vi "Example Modbus Slave.vi"() -> ()   [LabVIEW 2010]
uses:
  C:/tf/play/labview/Tinkerforge.dll
  Tinkerforge.dll
panel:
  out "registerValue":i32
  out "registerAddress":i64
  out "message":string
  out "requestID":u8
  in  "stop":bool
  in  "uid":string="amb"
  in  "port":i32=4223
  in  "host":string="localhost"
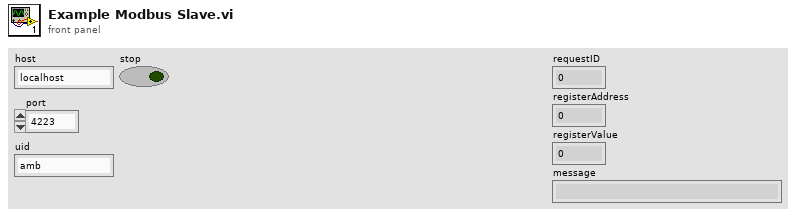
[diagram p1: front panel]
types:
  T1 = cluster{"requestID":u8, "registerAddress":i64, "registerValue":i32}
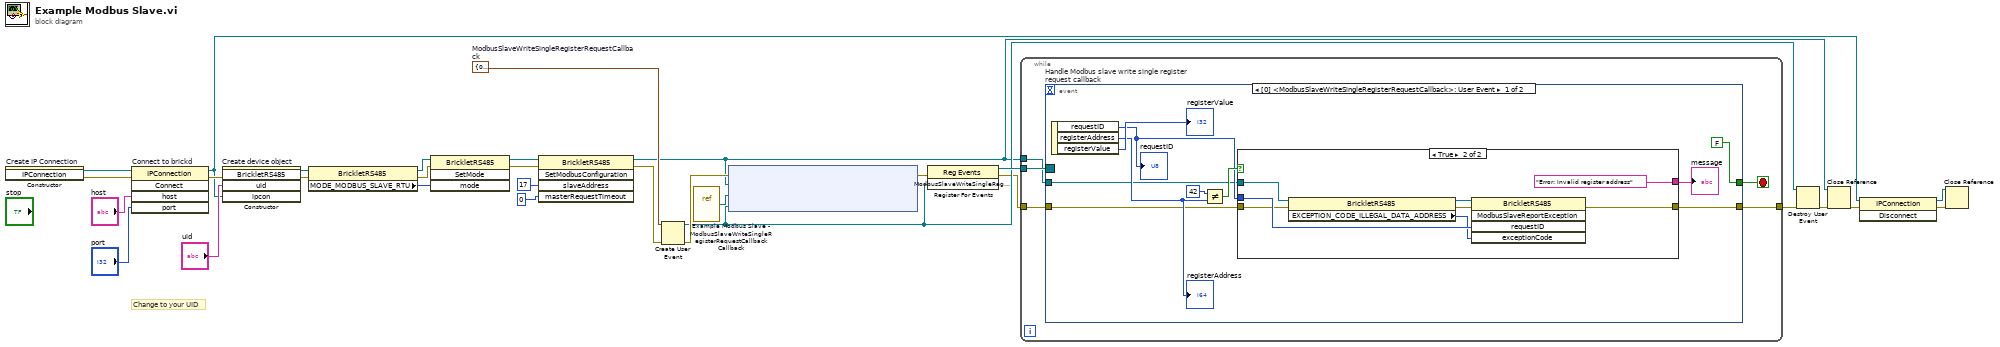
[diagram p0: block diagram]
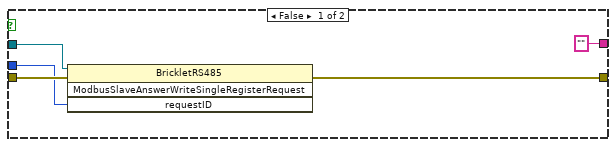
[diagram p2: hidden frame]
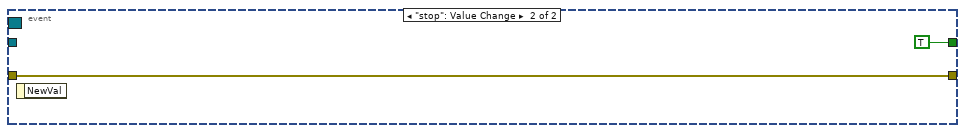
[diagram p3: hidden frame]
diagram:
  w14 = T1 {"requestID"=0, "registerAddress"=0, "registerValue"=0}  # ModbusSlaveWriteSingleRegisterRequestCallback
  # "Change to your UID"
  n1 = constructor on="Create IP Connection" class="IPConnection"() -> (reference out=w30:refnum<k24>, error out=w15:errorcluster)  [unwired: 3 in, 1 out]
  n2 = invoke on="Connect to brickd" class="IPConnection" method="Connect"(reference=w30, error in=w15, "host"="host", "port"="port") -> (reference out=w23:refnum<k24>, error out=w26:errorcluster)  [unwired: 1 in, 3 out]
  n3 = constructor on="Create device object" class="BrickletRS485"(error in=w26, "uid"="uid", "ipcon"=w23) -> (reference out=w13:refnum<k24>, error out=w12:errorcluster)  [unwired: 2 in, 3 out]
  n4 = property class="BrickletRS485"(reference=w13, error in=w12) -> (reference out=w10:refnum<k24>, error out=w11:errorcluster, "MODE_MODBUS_SLAVE_RTU"=w9:u8)
  n5 = invoke class="BrickletRS485" method="SetMode"(reference=w10, error in=w11, "mode"=w9) -> (reference out=w8:refnum<k24>, error out=w6:errorcluster)  [unwired: 1 in, 2 out]
  n6 = invoke class="BrickletRS485" method="SetModbusConfiguration"(reference=w8, error in=w6, "slaveAddress"=u8 17, "masterRequestTimeout"=i64 0) -> (reference out=w1:refnum<k24>, error out=w7:errorcluster)  [unwired: 1 in, 3 out]
  n7 = Create User Event(user event datatype=w14, error in=w7) -> (user event=w17:refnum<user-event>, error out=w21:errorcluster)
  n8 = vi-ref "Example Modbus Slave - ModbusSlaveWriteSingleRegisterRequestCallback Callback.vi"() -> ("vi reference"=w2:refnum<vi>)
  n9 = node ("Register Event Callback")(w21, w1, w2, w17) -> (w20:errorcluster)  [unwired: 1 in, 1 out]
  n10 = register-events(error in=w20, w17) -> (reference out=w19:refnum<event-registration>, error out=w3:errorcluster)  [unwired: 1 in]
  n11 = while {
    tunnel: w19 -> [w32]
    tunnel: [w35] -> w18
    tunnel: w3 -> [w34]
    tunnel: w1 -> [w31]
    stop <- w33 stop-if-true
    n12 = event "Handle Modbus slave write single register request callback" shown="[0] <ModbusSlaveWriteSingleRegisterRequestCallback>: User Event" {
      selector: w32 -> [_ _]
      dyn-events: _ -> [_ _]
      timeout: _ -> [_ _]
      tunnel: [w38 w59] -> w35
      tunnel: w34 -> [w39 w59]
      tunnel: [FALSE TRUE] -> w33
      tunnel: w31 -> [w36 _]
      event User Event {
        n13 = event-data() -> ("requestID"=w37:u8, "registerAddress"=w43:i64, "registerValue"=→"registerValue":i32)  [unwired: 1 in]
        "requestID" <- w37
        "registerAddress" <- w43
        n14 = Not Equal?(x=i64 42, y=w43) -> (x != y?=w41:bool)
        n15 = case shown="True" w41 {
          tunnel: ["" ("f") "Error: Invalid register address"] -> w40
          tunnel: w39 -> [w48 w54]
          tunnel: [w46 w57] -> w38
          tunnel: w37 -> [w47 w56]
          tunnel: w36 -> [w49 w55]
          frame False {
            n16 = invoke class="BrickletRS485" method="ModbusSlaveAnswerWriteSingleRegisterRequest"(reference=w49, error in=w48, "requestID"=w47) -> (error out=w46:errorcluster)  [unwired: 1 in, 3 out]
          }
          frame True {
            n17 = property class="BrickletRS485"(reference=w55, error in=w54) -> (reference out=w52:refnum<k24>, error out=w53:errorcluster, "EXCEPTION_CODE_ILLEGAL_DATA_ADDRESS"=w51:i16)
            n18 = invoke class="BrickletRS485" method="ModbusSlaveReportException"(reference=w52, error in=w53, "requestID"=w56, "exceptionCode"=w51) -> (error out=w57:errorcluster)  [unwired: 1 in, 4 out]
          }
        }
        "message" <- w40
      }
      event "stop": Value Change {
        n19 = event-data() -> ()  [unwired: 1 in, 1 out]
      }
    }
  }
  n20 = Destroy User Event(user event=w17, error in=w18) -> (error out=w16:errorcluster)
  n21 = Close Reference(reference=w1, error in (no error)=w16) -> (error out=w25:errorcluster)
  n22 = invoke class="IPConnection" method="Disconnect"(reference=w23, error in=w25) -> (reference out=w22:refnum<k24>, error out=w24:errorcluster)  [unwired: 1 in, 1 out]
  n23 = Close Reference(reference=w22, error in (no error)=w24) -> ()  [unwired: 1 out]
